vi "writtenevenoddfunc.vi"(1 "Numeric":dbl) -> (0 "concatenated string":string)   [LabVIEW 2019]
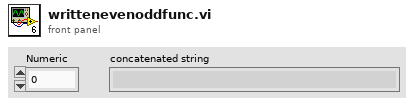
[diagram p1: front panel]
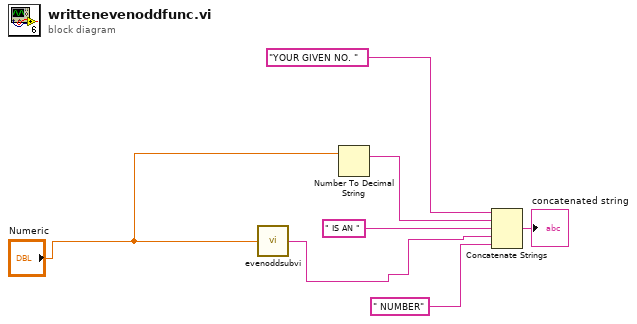
[diagram p0: block diagram]
diagram:
  n1 = call "evenoddsubvi.vi"("x"="Numeric") -> ("s? t:f"=w5:string)
  n2 = Number To Decimal String(number="Numeric") -> (decimal integer string=w3:string)  [unwired: 1 in]
  n3 = Concatenate Strings("YOUR GIVEN NO. " ("string"), w3, " IS AN " ("string"), w5, " NUMBER" ("string")) -> (→"concatenated string":string)
